vi "ASCII to Blowfish Encrypted.vi"() -> ()   [LabVIEW 2018, in "BNT_Factories.lvlib"]
doc: "Read ASCII file, encrypt using blowfish and write to filename.bf."
uses:
  BNT_Factories.lvlib
panel:
  out "Error Out":errorcluster
  in  "Password":string
  in  "CSPP-Ini-File":path
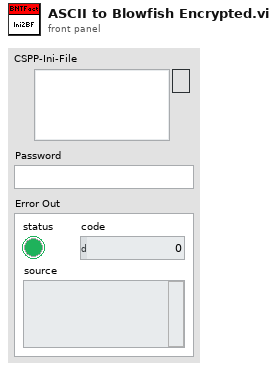
[diagram p1: front panel]
types:
  T1 = enum16{"open", "replace", "create", "open or create", "replace or create", "replace or create with confirmation"}
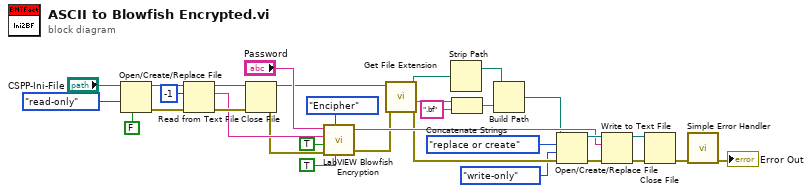
[diagram p0: block diagram]
diagram:
  n1 = Open/Create/Replace File(file path (use dialog)="CSPP-Ini-File", access (0:read/write)=enum16{"read/write", "read-only", "write-only"}."read-only", disable buffering (F)=FALSE) -> (refnum out=w31:refnum<file>, error out=w30:errorcluster)  [unwired: 3 in, 1 out]
  n2 = Read from Text File(file (use dialog)=w31, count=-1, error in=w30) -> (refnum out=w28:refnum<file>, text=w25:string, error out=w29:errorcluster)  [unwired: 1 in, 1 out]
  n3 = Close File(refnum=w28, error in=w29) -> (path=w13:path, error out=w10:errorcluster)
  n4 = call <userlib>:"LabVIEW Blowfish Encryption.vi"("Password"="Password", "Enc/Dec"=enum16{"Encipher", "Decipher"}."Encipher", "Input Text"=w25, "Compress Before\n encrypting?"=TRUE ("Compress Before\n encrypting?"), "Output As ASCII\nfor email Transmission"=TRUE ("Output As ASCII\nfor email Transmission"), "error in (no error)"=w10) -> ("Output text"=w20:string, "error out"=w9:errorcluster)  [unwired: 1 out]
  n5 = call <vilib>:"Get File Extension.vi"("error in (no error)"=w9, "file"=w13) -> ("error out"=w8:errorcluster, "filename without extension"=w12:string, "dup file"=w7:path)  [unwired: 5 in, 2 out]
  n6 = Strip Path(path=w7) -> (stripped path=w6:path)  [unwired: 1 out]
  n7 = Concatenate Strings(w12, ".bf" ("string")) -> (w5:string)
  n8 = Build Path(base path=w6, name or relative path=w5) -> (appended path=w4:path)
  n9 = Open/Create/Replace File(file path (use dialog)=w4, error in=w8, operation (0:open)=T1."replace or create", access (0:read/write)=enum16{"read/write", "read-only", "write-only"}."write-only") -> (refnum out=w22:refnum<file>, error out=w21:errorcluster)  [unwired: 2 in, 1 out]
  n10 = Write to Text File(file (use dialog)=w22, text=w20, error in=w21) -> (refnum out=w19:refnum<file>, error out=w18:errorcluster)  [unwired: 1 in, 1 out]
  n11 = Close File(refnum=w19, error in=w18) -> (error out=w3:errorcluster)  [unwired: 1 out]
  n12 = call <vilib>:"Simple Error Handler.vi"("error in (no error)"=w3) -> ("error out"=→"Error Out":errorcluster)  [unwired: 4 in, 4 out]
